vi "Get_Averages.vi"(8 "error in (no error)":errorcluster, 11 "VISA resource name":refnum<visa-resource-name>="Master_Oscilloscope") -> (0 "error out":errorcluster, 1 "Averages":string[](array[string]), 2 "number":i32, 3 "VISA resource name out":refnum<visa-resource-name>)   [LabVIEW 2020]
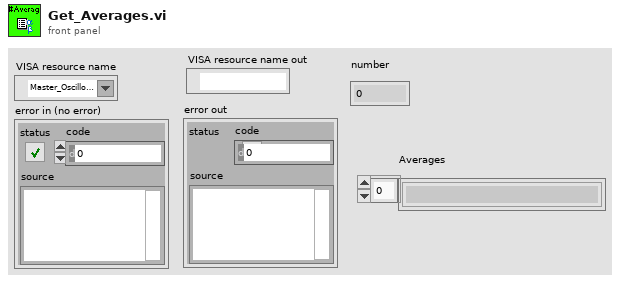
[diagram p1: front panel]
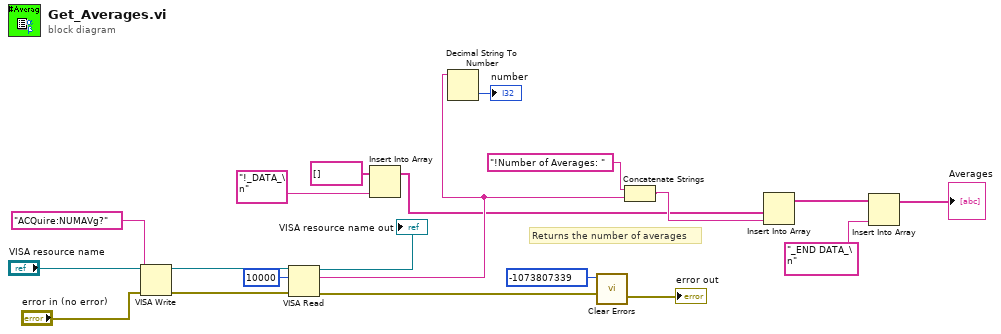
[diagram p0: block diagram]
diagram:
  # "Returns the number of averages"
  n1 = VISA Write(VISA resource name="VISA resource name", write buffer="ACQuire:NUMAVg?", error in (no error)="error in (no error)") -> (VISA resource name out=w20:refnum<visa-resource-name>, error out=w19:errorcluster)  [unwired: 1 out]
  n2 = VISA Read(VISA resource name=w20, byte count=u32 10000, error in (no error)=w19) -> (VISA resource name out=→"VISA resource name out":refnum<visa-resource-name>, read buffer=w8:string, error out=w10:errorcluster)  [unwired: 1 out]
  n3 = Insert Into Array(array=string[] [], new element="!_DATA_\n") -> (w4:string[])  [unwired: 1 in]
  n4 = Decimal String To Number(string=w8) -> (number=→"number":i32)  [unwired: 2 in, 1 out]
  n5 = call <vilib>:"Clear Errors.vi"("error in (no error)"=w10, "specific error code to clear (0: all)"=-1073807339) -> ("error out"=→"error out":errorcluster)  [unwired: 4 in, 1 out]
  n6 = Concatenate Strings("!Number of Averages: ", w8) -> (w7:string)
  n7 = Insert Into Array(array=w4, new element=w7) -> (w3:string[])  [unwired: 1 in]
  n8 = Insert Into Array(array=w3, new element="_END DATA_\n" ("new element/subarray")) -> (→"Averages":string[])  [unwired: 1 in]
